vi "IR LIDAR.vi"() -> (0 "error out":errorcluster, 3 "Range":T1)   [LabVIEW 2014]
uses:
  <vilib>/myRIO/Instrument Drivers/Onboard IO/AI/typedefs/AI Reference.ctl
  <vilib>/myRIO/Common/Instrument Driver Framework/Utilities/typedefs/myRIO Generic Hardware Reference.ctl
  <vilib>/myRIO/Common/Instrument Driver Framework/Utilities/typedefs/Hardware Version Enum.ctl
  <vilib>/myRIO/Common/Instrument Driver Framework/Utilities/typedefs/myRIO v1.0 Reference.ctl
  <vilib>/myRIO/Common/Instrument Driver Framework/Utilities/typedefs/Generic FPGA Reference.ctl
  <vilib>/myRIO/Common/Instrument Driver Framework/myRIO v1.0/AI/typedefs/AI Channels List.ctl
  <vilib>/myRIO/Common/Instrument Driver Framework/myRIO v1.0/AI/typedefs/AI Channels Enum.ctl
  <vilib>/myRIO/Common/Instrument Driver Framework/Utilities/typedefs/Analog Scaling Constants List.ctl
  <vilib>/myRIO/Common/Instrument Driver Framework/Utilities/typedefs/Analog Scaling Constants.ctl
  <vilib>/userdefined/High Color/nirio_resource_hc.ctl
  <vilib>/myRIO/Common/Instrument Driver Framework/Utilities/vis/Is FPGA Ref Available.vi
  <vilib>/myRIO/Common/Instrument Driver Framework/myRIO v1.0/AI/vis/myRIO v1.1 Open AI.vi
  <vilib>/myRIO/Instrument Drivers/Onboard IO/AI/vis/Read.vi
  <vilib>/myRIO/Common/Instrument Driver Framework/Utilities/vis/Validate Channels.vi
  <vilib>/myRIO/Common/Instrument Driver Framework/myRIO v1.0/AI/vis/myRIO v1.0 Reserve AI.vi
  <vilib>/myRIO/Common/Instrument Driver Framework/myRIO v1.0/AI/vis/myRIO v1.0 Build MUX Configuration AI.vi
  <vilib>/myRIO/Common/Instrument Driver Framework/myRIO v1.0/Resource Manager/vis/myRIO v1.0 Reserve Channel List.vi
  <vilib>/myRIO/Common/Instrument Driver Framework/myRIO v1.0/Resource Manager/vis/myRIO v1.0 Reserve Channel.vi
  <vilib>/myRIO/Common/Instrument Driver Framework/myRIO v1.0/Resource Manager/vis/myRIO v1.0 Unreserve Channel.vi
  <vilib>/myRIO/Common/Instrument Driver Framework/myRIO v1.0/Resource Manager/vis/myRIO v1.0 Build Mutex Name.vi
  <vilib>/Utility/VariantDataType/GetNumericInfo.vi
  <vilib>/Utility/error.llb/Error Cluster From Error Code.vi
  <vilib>/myRIO/Common/Instrument Driver Framework/myRIO v1.0/myRIO v1.1 Open.vi
  <vilib>/myRIO/Common/Instrument Driver Framework/myRIO v1.0/AI/vis/myRIO v1.0 Get Scaling Constants AI.vi
  <vilib>/myRIO/Common/Instrument Driver Framework/Utilities/vis/IO Manager.vi
  <vilib>/myRIO/Common/Instrument Driver Framework/Utilities/vis/Configuration Manager.vi
  <vilib>/myRIO/Common/Instrument Driver Framework/myRIO v1.0/myRIO v1.0 Close.vi
  <vilib>/myRIO/Common/Instrument Driver Framework/myRIO v1.0/AI/vis/myRIO v1.0 Read AI.vi
  <vilib>/myRIO/Express VI/Onboard IO/AI/AI Express VI.xnode
  <vilib>/myRIO/Instrument Drivers/Onboard IO/AI/vis/myRIO AI Open.xnode
  <vilib>/myRIO/Instrument Drivers/Onboard IO/AI/AI.lvlib
panel:
  # "This subVI reads and \ncalibrates the three\nSharp IR\nrange sensor"
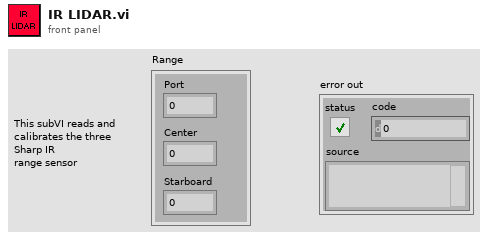
[diagram p1: front panel]
types:
  T1 = cluster{"Port":dbl, "Center":dbl, "Starboard":dbl}
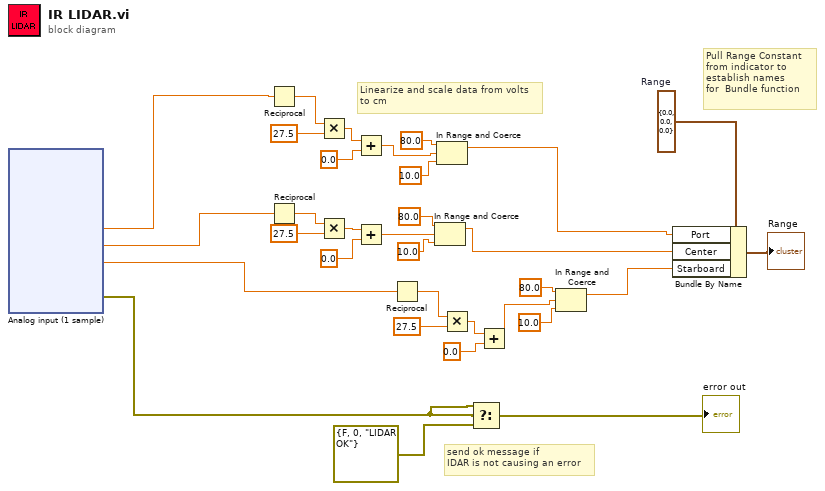
[diagram p0: block diagram]
diagram:
  w25 = T1 {"Port"=0.0, "Center"=0.0, "Starboard"=0.0}  # Range
  # "Linearize and scale data from volts\nto cm"
  # "Pull Range Constant\nfrom indicator to\nestablish names\nfor  Bundle function"
  # "send ok message if\nIDAR is not causing an error"
  n1 = xnode "Analog input (1 sample)"() -> ("Port Range (B/AI0 (Pin 3))"=w15:dbl, "Center Range (B/AI1 (Pin 5))"=w14:dbl, "Starboard Range (B/AI2 (Pin 7))"=w13:dbl, "error out"=w32:errorcluster)  [unwired: 1 in]
  n2 = Reciprocal(x=w15) -> (1/x=w26:dbl)
  n3 = Reciprocal(x=w14) -> (1/x=w23:dbl)
  n4 = Multiply(x=w26, y=27.5 ("Kscale [cm-V]")) -> (x*y=w29:dbl)
  n5 = Multiply(x=w23, y=27.5 ("Kscale [cm-V]")) -> (x*y=w20:dbl)
  n6 = Add(x=w29, y=0.0 ("Koffset [cm]")) -> (x+y=w12:dbl)
  n7 = Add(x=w20, y=0.0 ("Koffset [cm]")) -> (x+y=w8:dbl)
  n8 = Reciprocal(x=w13) -> (1/x=w16:dbl)
  n9 = In Range and Coerce(upper limit=80.0, x=w8, lower limit=10.0) -> (coerced(x)=w5:dbl)  [unwired: 1 out]
  n10 = In Range and Coerce(upper limit=80.0, x=w12, lower limit=10.0) -> (coerced(x)=w9:dbl)  [unwired: 1 out]
  n11 = Multiply(x=w16, y=27.5 ("Kscale [cm-V]")) -> (x*y=w19:dbl)
  n12 = Select(t=w32, s=w32, f=errorcluster {"status"=FALSE, "code"=0, "source"="LIDAR OK"} ("error out")) -> (s? t:f=→"error out":errorcluster)
  n13 = Add(x=w19, y=0.0 ("Koffset [cm]")) -> (x+y=w2:dbl)
  n14 = In Range and Coerce(upper limit=80.0, x=w2, lower limit=10.0) -> (coerced(x)=w1:dbl)  [unwired: 1 out]
  n15 = Bundle By Name "Bundle By Name"(cluster=w25, "Port"=w9, "Center"=w5, "Starboard"=w1) -> (→"Range":T1)
